vi "Update.vi"(7 "LabVIEW Web Service Request":refnum<class "Web Request.lvclass">) -> (3 "value":string)   [LabVIEW 2013]
uses:
  <vilib>/wsapi/Web Request.lvclass
  ACNET Monitor.lvlib
panel:
  in  "XML File Path":path=path "C:/Users/plane/Documents/acnet_monitor_config_from_acnetize.xml"
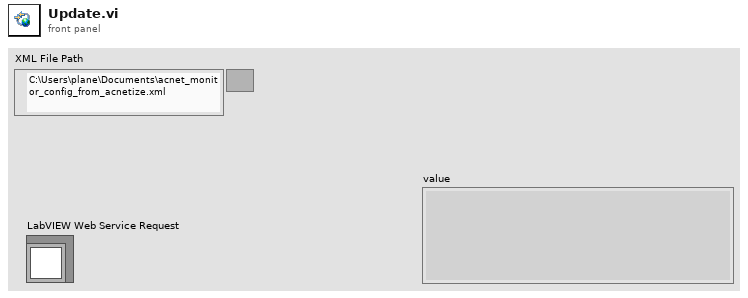
[diagram p1: front panel]
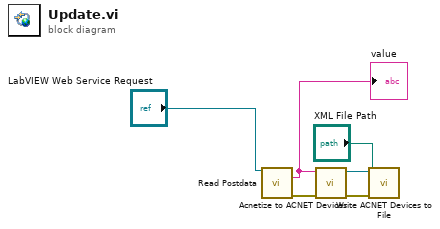
[diagram p0: block diagram]
diagram:
  n1 = call <vilib>:"Read Postdata.vi"("LabVIEW Web Service Request"="LabVIEW Web Service Request") -> ("postdata"=w5:string, "error out"=w4:errorcluster)  [unwired: 12 in, 1 out]
  "value" <- w5
  n2 = call "Acnetize to ACNET Devices.vi"("error in (no error)"=w4, "Acnetize Configuration"=w5) -> ("error out"=w2:errorcluster, "ACNET Devices"=w3:refnum<class "ACNET Devices.lvclass">)  [unwired: 8 in]
  n3 = call "Write ACNET Devices to File.vi"("error in (no error)"=w2, "XML File Path"="XML File Path", "ACNET Devices in"=w3) -> ()  [unwired: 7 in, 2 out]
